vi "PathPlanner_PathFinder_Cost.vi"(9 "sGoalLoc":T1, 11 "sStartLoc":T1) -> (3 "Cost":dbl)   [LabVIEW 2019]
uses:
  PathPlannerLib24/TypeDef/PathPlannerFinderGridPosition.ctl
  PathPlannerLib24/VI/PathPlanner_GridPosition_Get.vi
  PathPlannerLib24/VI/PathPlanner_GridPosition_New.vi
  PathPlannerLib24/VI/PathPlanner_GridPosition_Print.vi
  PathPlannerLib24/VI/PathPlanner_PathFinder_Globals.vi
  PathPlannerLib24/PathPlanner24.lvlib
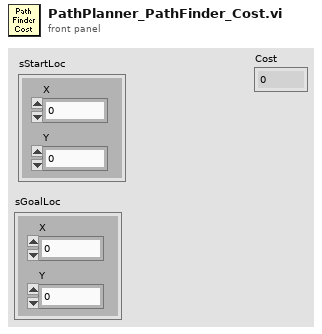
[diagram p1: front panel]
types:
  T1 = typedef "PathPlanner24.lvlib/PathPlannerFinderGridPosition.ctl" = cluster{"X":i32, "Y":i32}
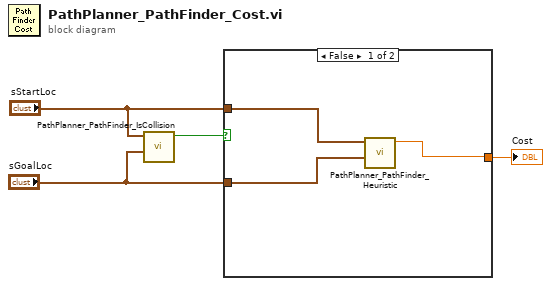
[diagram p0: block diagram]
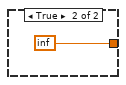
[diagram p2: hidden frame]
diagram:
  n1 = call "PathPlanner_PathFinder_IsCollision.vi"("sEnd"="sGoalLoc", "sStartLoc"="sStartLoc") -> ("Collision"=w3:bool)  [unwired: 9 in]
  n2 = case shown="False" w3 {
    tunnel: [w5 inf] -> w4
    tunnel: "sStartLoc" -> [w7 _]
    tunnel: "sGoalLoc" -> [w6 _]
    frame False {
      n3 = call "PathPlanner_PathFinder_Heuristic.vi"("sGoalLoc"=w6, "sStartLoc"=w7) -> ("heuristic"=w5:dbl)  [unwired: 9 in]
    }
    frame True {
    }
  }
  "Cost" <- w4
